vi "Change Panel.vi"(8 "error in (no error)":errorcluster, 10 "New Panel":refnum<class "Panel.lvclass">, 11 "Panel Actor in":refnum<class "Panel Actor.lvclass">) -> (0 "error out":errorcluster, 3 "Panel Actor out":refnum<class "Panel Actor.lvclass">)   [LabVIEW 2019, in "Panel Actor.lvlib" / "Panel Actor.lvclass"]
doc: "Changes the type of panel for the panel actor.\n\n----\nPlease see the following web address for additional documentation and tutorial information:\nhttp://www.mooregoodideas.com/mgi-panel-manager/\n\nAuthor: Derek Trepanier\n\nCopyright (c) 2018, Moore Good Ideas, Inc.\n\nAll rights reserved.\n\nRedistribution and use in source and binary forms, with or without modification, are permitted provided that the following conditions are met:\n\n * Redistributions of source code must retain the above copyright notice, this list of conditions and the following disclaimer.\n * Redistributions in binary form must reproduce the above copyright notice, this list of conditions and the following disclaimer in the documentation and/or other materials provided with the distribution.\n * Neither the name of Moore Good Ideas, Inc. nor the names of its contributors may be used to endorse or promote products derived from this software without specific prior written permission.\n\nTHIS SOFTWARE IS PROVIDED BY THE COPYRIGHT HOLDERS AND CONTRIBUTORS \"AS IS\" AND ANY EXPRESS OR IMPLIED WARRANTIES, INCLUDING, BUT NOT LIMITED TO, THE IMPLIED WARRANTIES OF MERCHANTABILITY AND FITNESS FOR A PARTICULAR PURPOSE ARE DISCLAIMED. IN NO EVENT SHALL THE COPYRIGHT OWNER OR CONTRIBUTORS BE LIABLE FOR ANY DIRECT, INDIRECT, INCIDENTAL, SPECIAL, EXEMPLARY, OR CONSEQUENTIAL DAMAGES (INCLUDING, BUT NOT LIMITED TO, PROCUREMENT OF SUBSTITUTE GOODS OR SERVICES; LOSS OF USE, DATA, OR PROFITS; OR BUSINESS INTERRUPTION) HOWEVER CAUSED AND ON ANY THEORY OF LIABILITY, WHETHER IN CONTRACT, STRICT LIABILITY, OR TORT (INCLUDING NEGLIGENCE OR OTHERWISE) ARISING IN ANY WAY OUT OF THE USE OF THIS SOFTWARE, EVEN IF ADVISED OF THE POSSIBILITY OF SUCH DAMAGE."
uses:
  Panel Actor.lvclass
  builds/Engine/Panel.lvlibp/Panel/Panel.lvclass
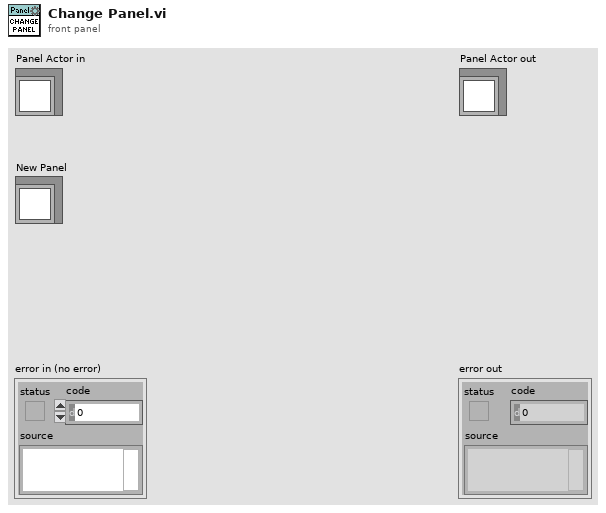
[diagram p1: front panel]
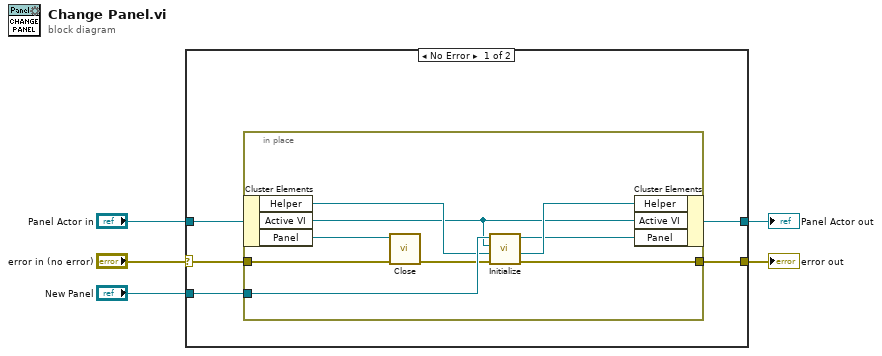
[diagram p0: block diagram]
diagram:
  n1 = case shown="No Error" "error in (no error)" {
    selector: "error in (no error)" -> [w7 w21]
    tunnel: [w6 w21] -> w4
    tunnel: [w9 w20] -> w2
    tunnel: "Panel Actor in" -> [w10 w20]
    tunnel: "New Panel" -> [w8 _]
    frame No Error {
      n2 = in-place {
        in-place-border: w8 -> [w19]
        in-place-border: w7 -> [w14]
        in-place-border: [w13] -> w6
        n3 = in-place-cluster #1(w10) -> ("Helper"=w17:refnum<class "Panel Helper.lvclass">, "Active VI"=w15:refnum<vi>, "Panel"=w11:refnum<class "Panel.lvclass">)
        n4 = call-dynamic "Close.vi"("Error In"=w14, "Panel In"=w11) -> ("Error Out"=w18:errorcluster)  [unwired: 9 in]
        n5 = call "Initialize.vi"("error in (no error)"=w18, "My Helper in"=w17, "VI Refnum"=w15, "Panel In"=w19) -> ("error out"=w13:errorcluster, "My Helper out"=w16:refnum<class "Panel Helper.lvclass">, "Panel Out"=w12:refnum<class "Panel.lvclass">)  [unwired: 5 in]
        n6 = in-place-cluster #1("Helper"=w16, "Active VI"=w15, "Panel"=w12) -> (w9:refnum<class "Panel Actor.lvclass">)
      }
    }
    frame Error {
    }
  }
  "error out" <- w4
  "Panel Actor out" <- w2
